vi "读取excel中所有表单数据.vi"(8 "错误输入（无错误）":errorcluster, 11 "excel路径":path) -> (0 "错误输出":errorcluster, 3 "所有表单数据":string[][][](array[string]))   [LabVIEW 2013, in "excel处理.lvlib"]
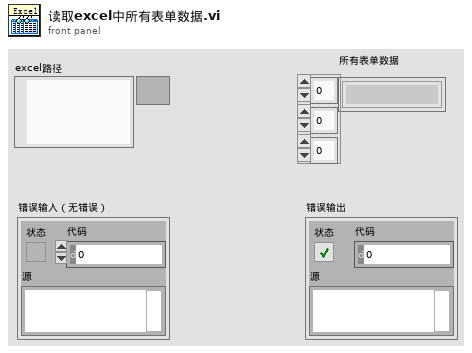
[diagram p1: front panel]
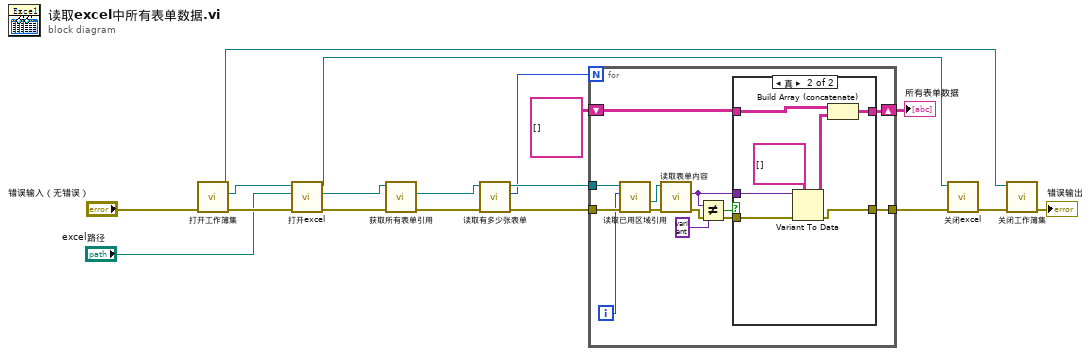
[diagram p0: block diagram]
diagram:
  n1 = call "打开工作簿集.vi"("错误输入（无错误）"="错误输入（无错误）") -> ("错误输出"=w18:errorcluster, "工作簿集"=w12:refnum<k7>, "excel.application输出"=w7:refnum<k7>)  [unwired: 8 in]
  n2 = call "打开excel.vi"("错误输入（无错误）"=w18, "excel路径"="excel路径", "工作簿引用"=w12) -> ("错误输出"=w17:errorcluster, "excel引用"=w11:refnum<k7>, "工作簿输出"=w8:refnum<k7>)  [unwired: 6 in]
  n3 = call "获取所有表单引用.vi"("错误输入（无错误）"=w17, "excel引用"=w11) -> ("错误输出"=w16:errorcluster, "Worksheets"=w10:refnum<k7>)  [unwired: 7 in, 1 out]
  n4 = call "读取有多少张表单.vi"("错误输入（无错误）"=w16, "所有表单引用"=w10) -> ("错误输出"=w15:errorcluster, "表单个数"=w6:i32, "所有表单引用输出"=w9:refnum<k7>)  [unwired: 7 in]
  n5 = for {
    N: w6 -> [_]
    tunnel: w15 -> [w30]
    tunnel: [w21] -> w14
    tunnel: w9 -> [w27]
    shift-right: [w20] -> w1
    shift-left: string[][][] [] -> [w19]
    i -> [w26]
    n6 = call "读取已用区域引用.vi"("错误输入（无错误）"=w30, "表单索引"=w26, "所有表单引用"=w27) -> ("错误输出"=w29:errorcluster, "选中引用输出"=w28:refnum<k7>)  [unwired: 5 in, 2 out]
    n7 = call "读取表单内容.vi"("错误输入（无错误）"=w29, "选中区域引用输入"=w28) -> ("错误输出"=w22:errorcluster, "数值"=w23:variant)  [unwired: 7 in, 1 out]
    n8 = Not Equal?(x=w23, y=variant) -> (x != y?=w24:bool)
    n9 = case shown="真" w24 {
      tunnel: w23 -> [_ w39]
      tunnel: w22 -> [w31 w38]
      tunnel: [w31 w37] -> w21
      tunnel: [w32 w34] -> w20
      tunnel: w19 -> [w32 w33]
      frame False {
      }
      frame True {
        n10 = Variant To Data(error in=w38, type=string[][] [], Variant=w39) -> (data=w35:string[][], error out=w37:errorcluster)
        n11 = Build Array (concatenate)(w33, w35) -> (w34:string[][][])
      }
    }
  }
  "所有表单数据" <- w1
  n12 = call "关闭excel.vi"("错误输入（无错误）"=w14, "引用"=w8) -> ("错误输出"=w13:errorcluster)  [unwired: 8 in, 1 out]
  n13 = call "关闭工作簿集.vi"("错误输入（无错误）"=w13, "工作薄引用"=w7) -> ("错误输出"=→"错误输出":errorcluster)  [unwired: 8 in, 1 out]
